vi "DAS240Main.vi"() -> ()   [LabVIEW 2016]
uses:
  <vilib>/NI/Modbus Library/API/Master/Modbus Master.lvclass
  C:/Program Files (x86)/National Instruments/LabVIEW 2016/vi.lib/NI/Modbus Library/API/Modbus API.lvclass
  <vilib>/NI/Modbus Library/API/Wrapper/Create TCP Master.vi
  <vilib>/Utility/file.llb/Write To Spreadsheet File (DBL).vi
  <vilib>/NI/Modbus Library/API/Wrapper/API Main.lvlib
panel:
  out "Logical channels":bool[](array[boolean])
  in  "CSV Delimiter":string=";"
  in  "File path":path
  in  "Record .CSV File?":bool
  out "Graphe déroulant":sgl(graph)
  in  "Waveform channel":i32
  in  "number of channels":u16=20
  in  "port (502)":u16=502
  in  "IP address":string="000.000.000.000"
  out "Channel values":sgl[](array[numeric])
  in  "stop":bool
  in  "update period (ms)":u32=100
  # "Modbus TCP Configuration"
  # "Update period"
  # "DataLogger Sefram DAS240 is a\nmultiplexed acquisition system.\nIt means that sampling frequency\ndepends on number of channel acquired\nand type of channel.\nUp to 60 channels, you should not set more\nthan 100 ms of update period."
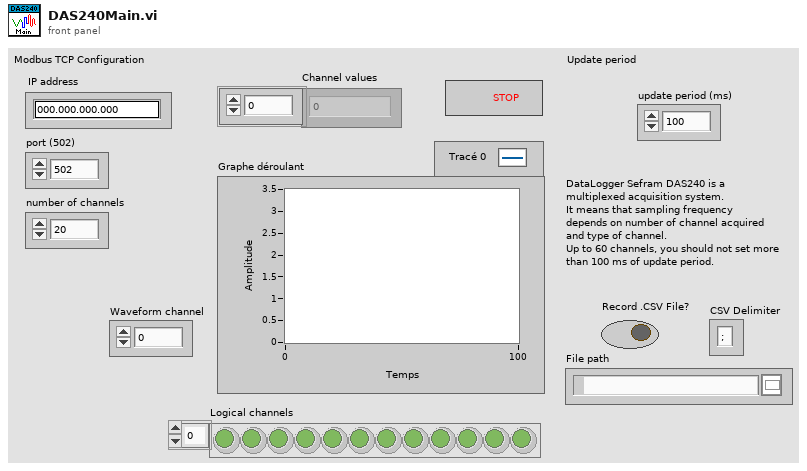
[diagram p1: front panel]
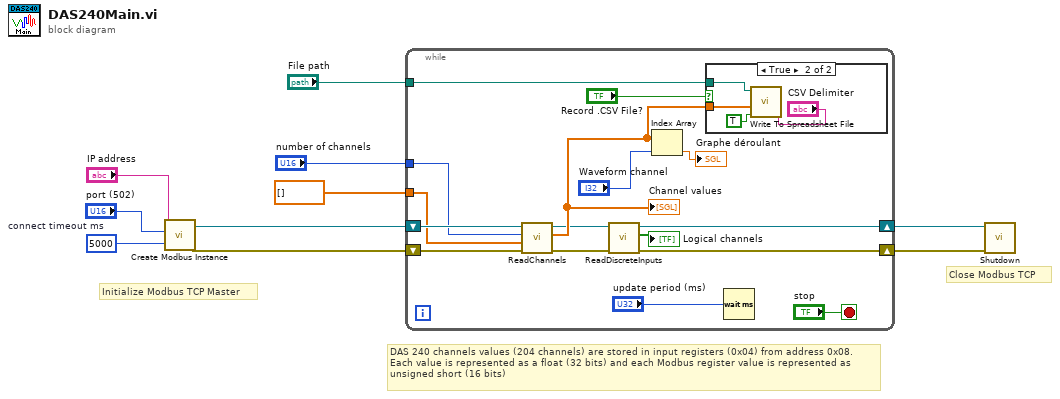
[diagram p0: block diagram]
diagram:
  w9 = 5000  # connect timeout ms
  # "DAS 240 channels values (204 channels) are stored in input registers (0x04) from address 0x08.\nEach value is represented as a float (32 bits) and each Modbus register value is represented as\nunsigned short (16 bits)"
  # "Close Modbus TCP"
  # "Initialize Modbus TCP Master"
  n1 = call-poly <vilib>:"Create Modbus Instance.vi"("connect timeout ms"=w9, "port (502)"="port (502)", "address"="IP address") -> ("error out"=w7:errorcluster, "TCP master instance"=w8:refnum<class "Modbus Master.lvclass">)  [unwired: 7 in]
  n2 = while {
    tunnel: sgl[] [] -> [w22]
    shift-right: [w12] -> w5
    shift-left: w7 -> [w23]
    shift-right: [w13] -> w6
    shift-left: w8 -> [w24]
    tunnel: "number of channels" -> [w21]
    tunnel: "File path" -> [w17]
    stop <- "stop" stop-if-true
    n3 = call "ReadChannels.vi"("error in"=w23, "Data in"=w22, "number of channels"=w21, "Modbus master in"=w24) -> ("error out"=w14:errorcluster, "Data out"=w16:sgl[], "Modbus master out"=w15:refnum<class "Modbus Master.lvclass">)  [unwired: 5 in]
    "Channel values" <- w16
    n4 = call "ReadDiscreteInputs.vi"("error in"=w14, "Modbus instance in"=w15) -> ("error out"=w12:errorcluster, "discrete inputs"=→"Logical channels":bool[], "Modbus instance out"=w13:refnum<class "Modbus Master.lvclass">)  [unwired: 7 in]
    n5 = Index Array(array=w16, index="Waveform channel") -> (element=→"Graphe déroulant":sgl)
    n6 = case shown="True" "Record .CSV File?" {
      tunnel: w17 -> [_ w30]
      tunnel: w16 -> [_ w29]
      frame False {
      }
      frame True {
        n7 = call-poly <vilib>:"Write To Spreadsheet File.vi"("delimiter (\\t)"="CSV Delimiter", "append to file? (new file:F)"=TRUE, "1D data"=w29, "file path (dialog if empty)"=w30) -> ()  [unwired: 4 in, 1 out]
      }
    }
    n8 = Wait (ms)(milliseconds to wait="update period (ms)") -> ()  [unwired: 1 out]
  }
  n9 = call-dynamic "Shutdown.vi"("error in"=w5, "Modbus master in"=w6) -> ()  [unwired: 9 in, 1 out]
